vi "PicoScope5000aClose.vi"(0 "handle":i16) -> ()   [LabVIEW 2020]
doc: "This closes the oscilloscope and should be called before exiting an application."
uses:
  ps5000a.dll
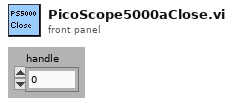
[diagram p1: front panel]
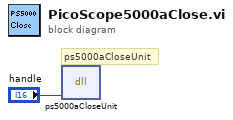
[diagram p0: block diagram]
diagram:
  # "ps5000aCloseUnit"
  n1 = dll-call lib="ps5000a.dll" fn="ps5000aCloseUnit" ("ps3000.dll:_ps3000_open_unit@0")("handle"="handle") -> ()  [unwired: 5 in, 2 out]
